vi "Vocal Efficiency Calc.vi"(3 "Pressure":waveform(dbl), 4 "SPL":dbl, 5 "Flow":waveform(dbl)) -> (1 "Vocal Efficiency":dbl)   [LabVIEW 2019, in "SubVIs.lvlib"]
uses:
  SubVIs.lvlib
  <vilib>/measure/madcrms.llb/Basic Averaged DC-RMS for 1 Chan.vi
  <vilib>/measure/NI_MAPro.lvlib
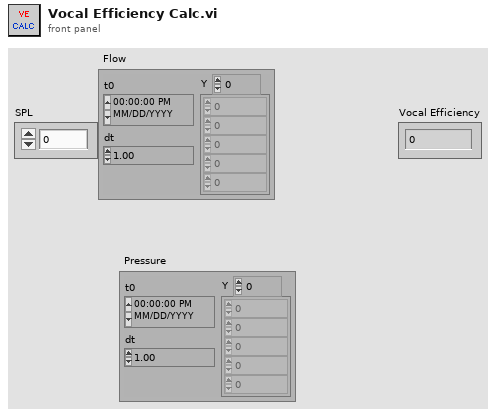
[diagram p1: front panel]
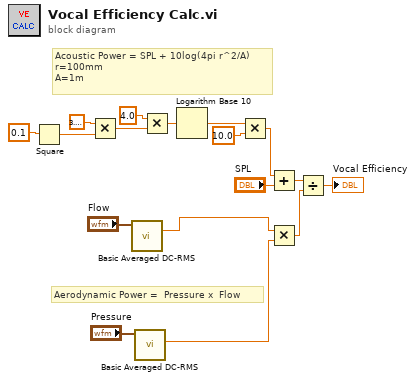
[diagram p0: block diagram]
diagram:
  # "Aerodynamic Power =  Pressure x  Flow"
  # "Acoustic Power = SPL + 10log(4pi r^2/A)\nr=100mm\nA=1m"
  n1 = Square(x=0.1) -> (x^2=w14:dbl)
  n2 = Multiply(x=3.141592653589793, y=w14) -> (x*y=w12:dbl)
  n3 = call-poly <vilib>:"Basic Averaged DC-RMS.vi"("signal in"="Flow") -> ("RMS value"=w1:dbl)  [unwired: 7 in, 3 out]
  n4 = call-poly <vilib>:"Basic Averaged DC-RMS.vi"("signal in"="Pressure") -> ("RMS value"=w2:dbl)  [unwired: 7 in, 3 out]
  n5 = Multiply(x=4.0, y=w12) -> (x*y=w10:dbl)
  n6 = Logarithm Base 10(1:w10) -> (0:w17:dbl)
  n7 = Multiply(x=w17, y=10.0) -> (x*y=w9:dbl)
  n8 = Add(x=w9, y="SPL") -> (x+y=w7:dbl)
  n9 = Multiply(x=w1, y=w2) -> (x*y=w6:dbl)
  n10 = Divide(x=w7, y=w6) -> (x/y=→"Vocal Efficiency":dbl)
